vi "ADIS16448_RoboRIO_Teensy_GetData.vi"(0 "SerialPortRefIn":T3, 11 "error in":errorcluster) -> (4 "SerialPortRefOut":T3, 6 "IMU Angles Out":T2, 8 "IMU AHRS Out":cluster{"Pitch":dbl, "Roll":dbl, "Yaw":dbl}, 10 "IMU Instant Out":T1, 15 "error out":errorcluster)   [LabVIEW 2016, in "ADIS16448-Teensy.lvlib"]
uses:
  ADIS16448-Teensy.lvlib
  <vilib>/Rock Robotics/WPI/SerialPort/WPI_SerialPortRef.ctl
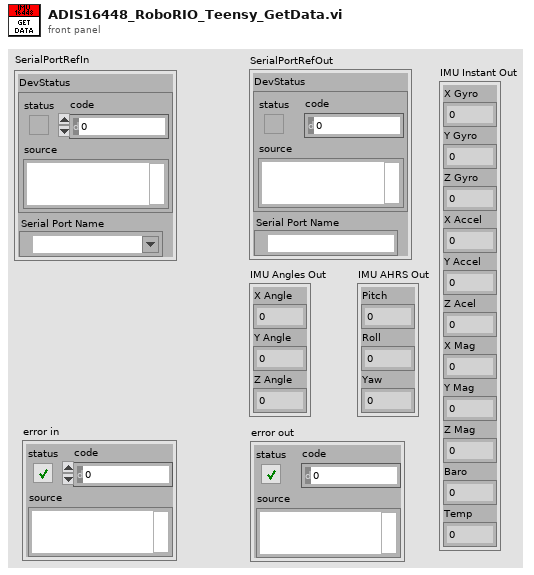
[diagram p1: front panel]
types:
  T1 = cluster{"X Gyro":dbl, "Y Gyro":dbl, "Z Gyro":dbl, "X Accel":dbl, "Y Accel":dbl, "Z Acel":dbl, "X Mag":dbl, "Y Mag":dbl, "Z Mag":dbl, "Baro":dbl, "Temp":dbl}
  T2 = cluster{"X Angle":dbl, "Y Angle":dbl, "Z Angle":dbl}
  T3 = typedef "WPI_SerialPortRef.ctl" = cluster{"DevStatus":errorcluster, "Serial Port Name":refnum<visa-resource-name>}
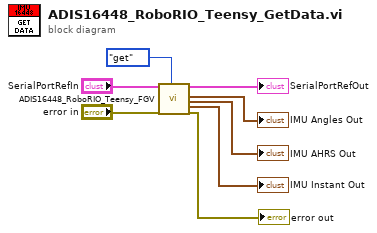
[diagram p0: block diagram]
diagram:
  n1 = call "ADIS16448_RoboRIO_Teensy_FGV.vi"("SerialPortRefIn"="SerialPortRefIn", "error in"="error in", "Operation"=enum16{"set", "get", "set reset"}."get") -> ("SerialPortRefOut"=→"SerialPortRefOut":T3, "IMU Angles Out"=→"IMU Angles Out":T2, "IMU AHRS Out"=→"IMU AHRS Out":cluster{"Pitch":dbl, "Roll":dbl, "Yaw":dbl}, "IMU Instant Out"=→"IMU Instant Out":T1, "error out"=→"error out":errorcluster)  [unwired: 10 in, 2 out]
